vi "Error Eater.vi"(2 "error in (no error)":errorcluster) -> ()   [LabVIEW 2020]
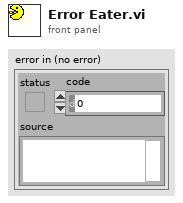
[diagram p1: front panel]
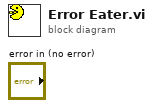
[diagram p0: block diagram]
diagram:
